vi "Get Virtual Instrument Configuration.vi"(8 "Error In":errorcluster, 10 "Virtual Instrument Identifier":string) -> (0 "Error Out":errorcluster, 1 "Virtual Instrument Configuration":refnum<class "Config from JSON.lvclass">, 2 "Found":bool)   [LabVIEW 2024, in "Instrument Manager.lvclass"]
uses:
  Instrument Manager.lvclass
  Config from JSON/Config from JSON.lvclass
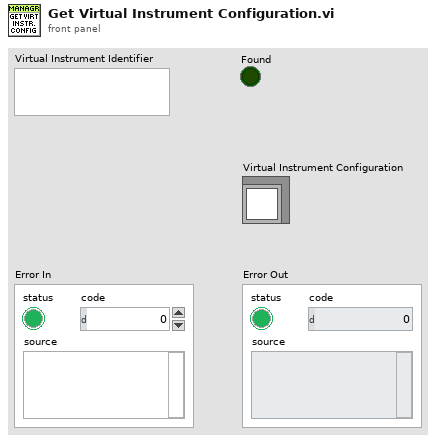
[diagram p1: front panel]
types:
  T1 = typedef "Instrument Manager.lvclass/ObjectAttributes.ctl" = cluster{"IInstruments":map{string, refnum<class "IInstrument.lvclass">}, "IVirtual Instruments":map{string, refnum<class "IVirtual Instrument.lvclass">}, "Instrument Configurations":map{string, refnum<class "Config from JSON.lvclass">}, "Virtual Instrument Configurations":map{string, refnum<class "Config from JSON.lvclass">}, "Action Point Configurations":map{string, refnum<class "Config from JSON.lvclass">}, "Action Points":map{string, refnum<class "Action Point.lvclass">}}
  T2 = map{string, refnum<class "Config from JSON.lvclass">}
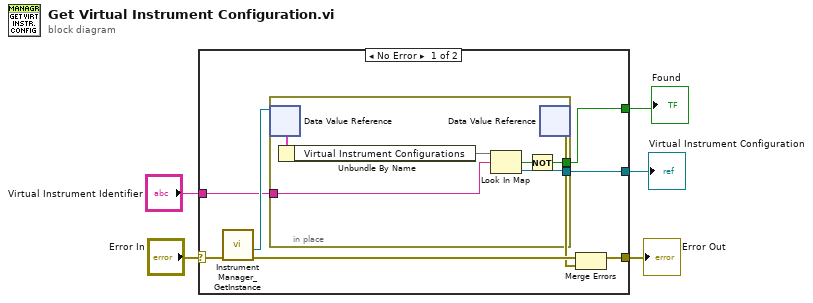
[diagram p0: block diagram]
diagram:
  n1 = case shown="No Error" "Error In" {
    selector: "Error In" -> [w13 w20]
    tunnel: [w11 w20] -> w4
    tunnel: [w9 _] -> w2
    tunnel: "Virtual Instrument Identifier" -> [w7 _]
    tunnel: [w6 _] -> w1
    frame No Error {
      n2 = call "Instrument Manager_GetInstance.vi"("Error In"=w13) -> ("Error Out"=w12:errorcluster, "DVRRefOut"=w8:refnum<data-value>)  [unwired: 6 in, 3 out]
      n3 = in-place {
        in-place-border: [w16] -> w9
        in-place-border: w7 -> [w17]
        in-place-border: [w14] -> w6
        n4 = in-place-dvr #1(w8) -> (w19:T1)  [unwired: 1 out]
        n5 = Unbundle By Name(w19) -> ("Virtual Instrument Configurations"=w18:T2)
        n6 = Look In Map(map=w18, key=w17) -> (key not found?=w15:bool, value=w16:refnum<class "Config from JSON.lvclass">)  [unwired: 1 in]
        n7 = Not(x=w15) -> (.not. x?=w14:bool)
        n8 = in-place-dvr #1() -> (w10:errorcluster)  [unwired: 1 in, 1 out]
      }
      n9 = Merge Errors(w12, w10) -> (w11:errorcluster)
    }
    frame Error {
    }
  }
  "Error Out" <- w4
  "Virtual Instrument Configuration" <- w2
  "Found" <- w1
